vi "16DUT Plot Subvi Ver1.0.vi"(6 "Plot":T1(ring), 7 "No of Rows":i32=10496, 8 "error in (no error)":errorcluster, 9 "WS1050/51":bool=TRUE, 10 "Bank":enum16{"C1", "C2", "C3"}(ring), 11 "file path (dialog if empty)":path) -> (0 "error out":errorcluster, 3 "Delta C_Min Plot":dbl[][](graph) caption="(Y) Multi Plot 2")   [LabVIEW 2012]
uses:
  <vilib>/Utility/file.llb/Read From Spreadsheet File (string).vi
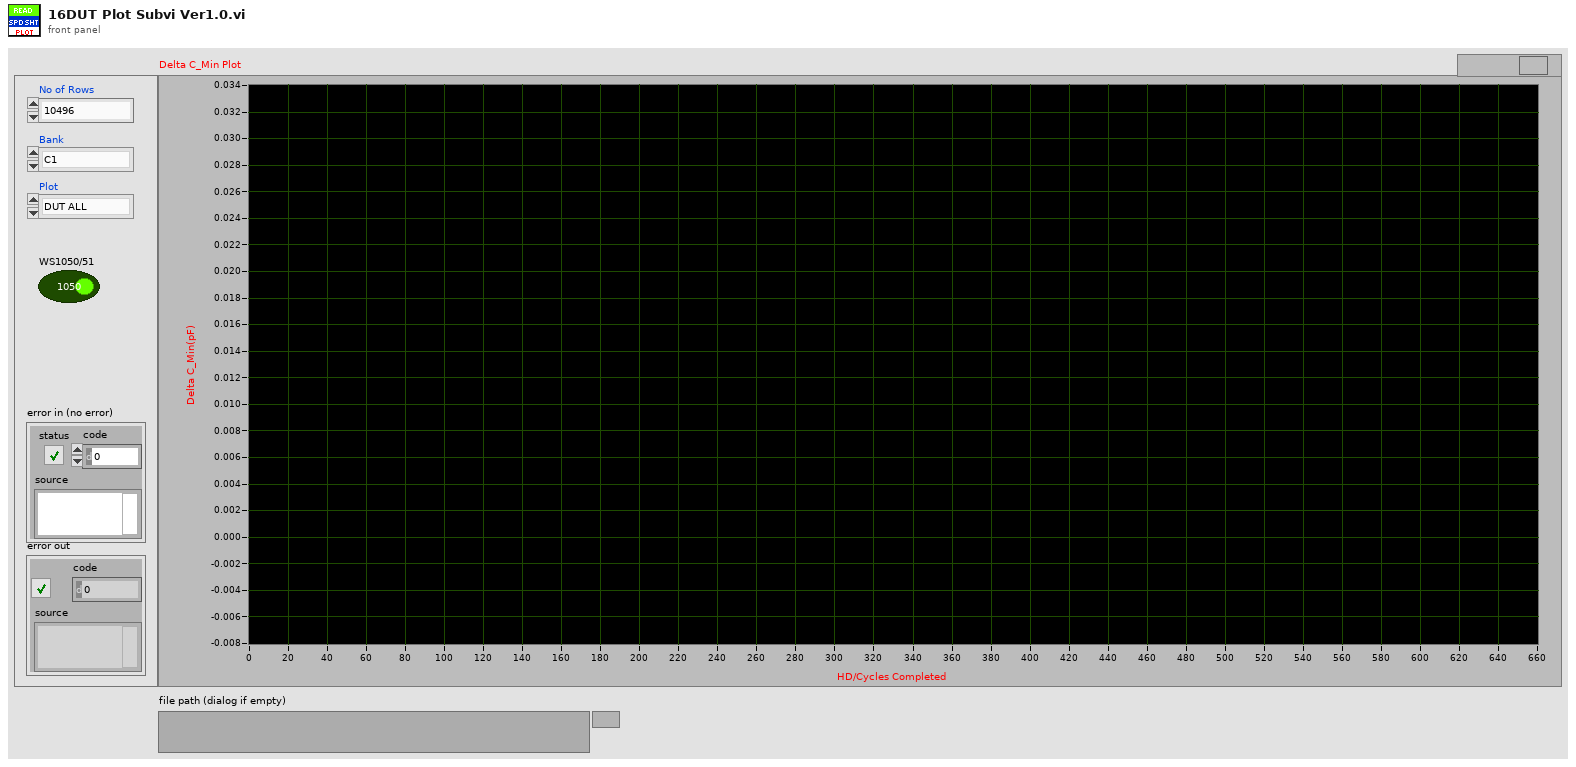
[diagram p1: front panel]
types:
  T1 = enum16{"DUT ALL", "DUT 01", "DUT 02", "DUT 03", "DUT 04", "DUT 05", "DUT 06", "DUT 07", "DUT 08", "DUT 09", "DUT 10", "DUT 11", "DUT 12", "DUT 13", "DUT 14", "DUT 15", "DUT 16"}
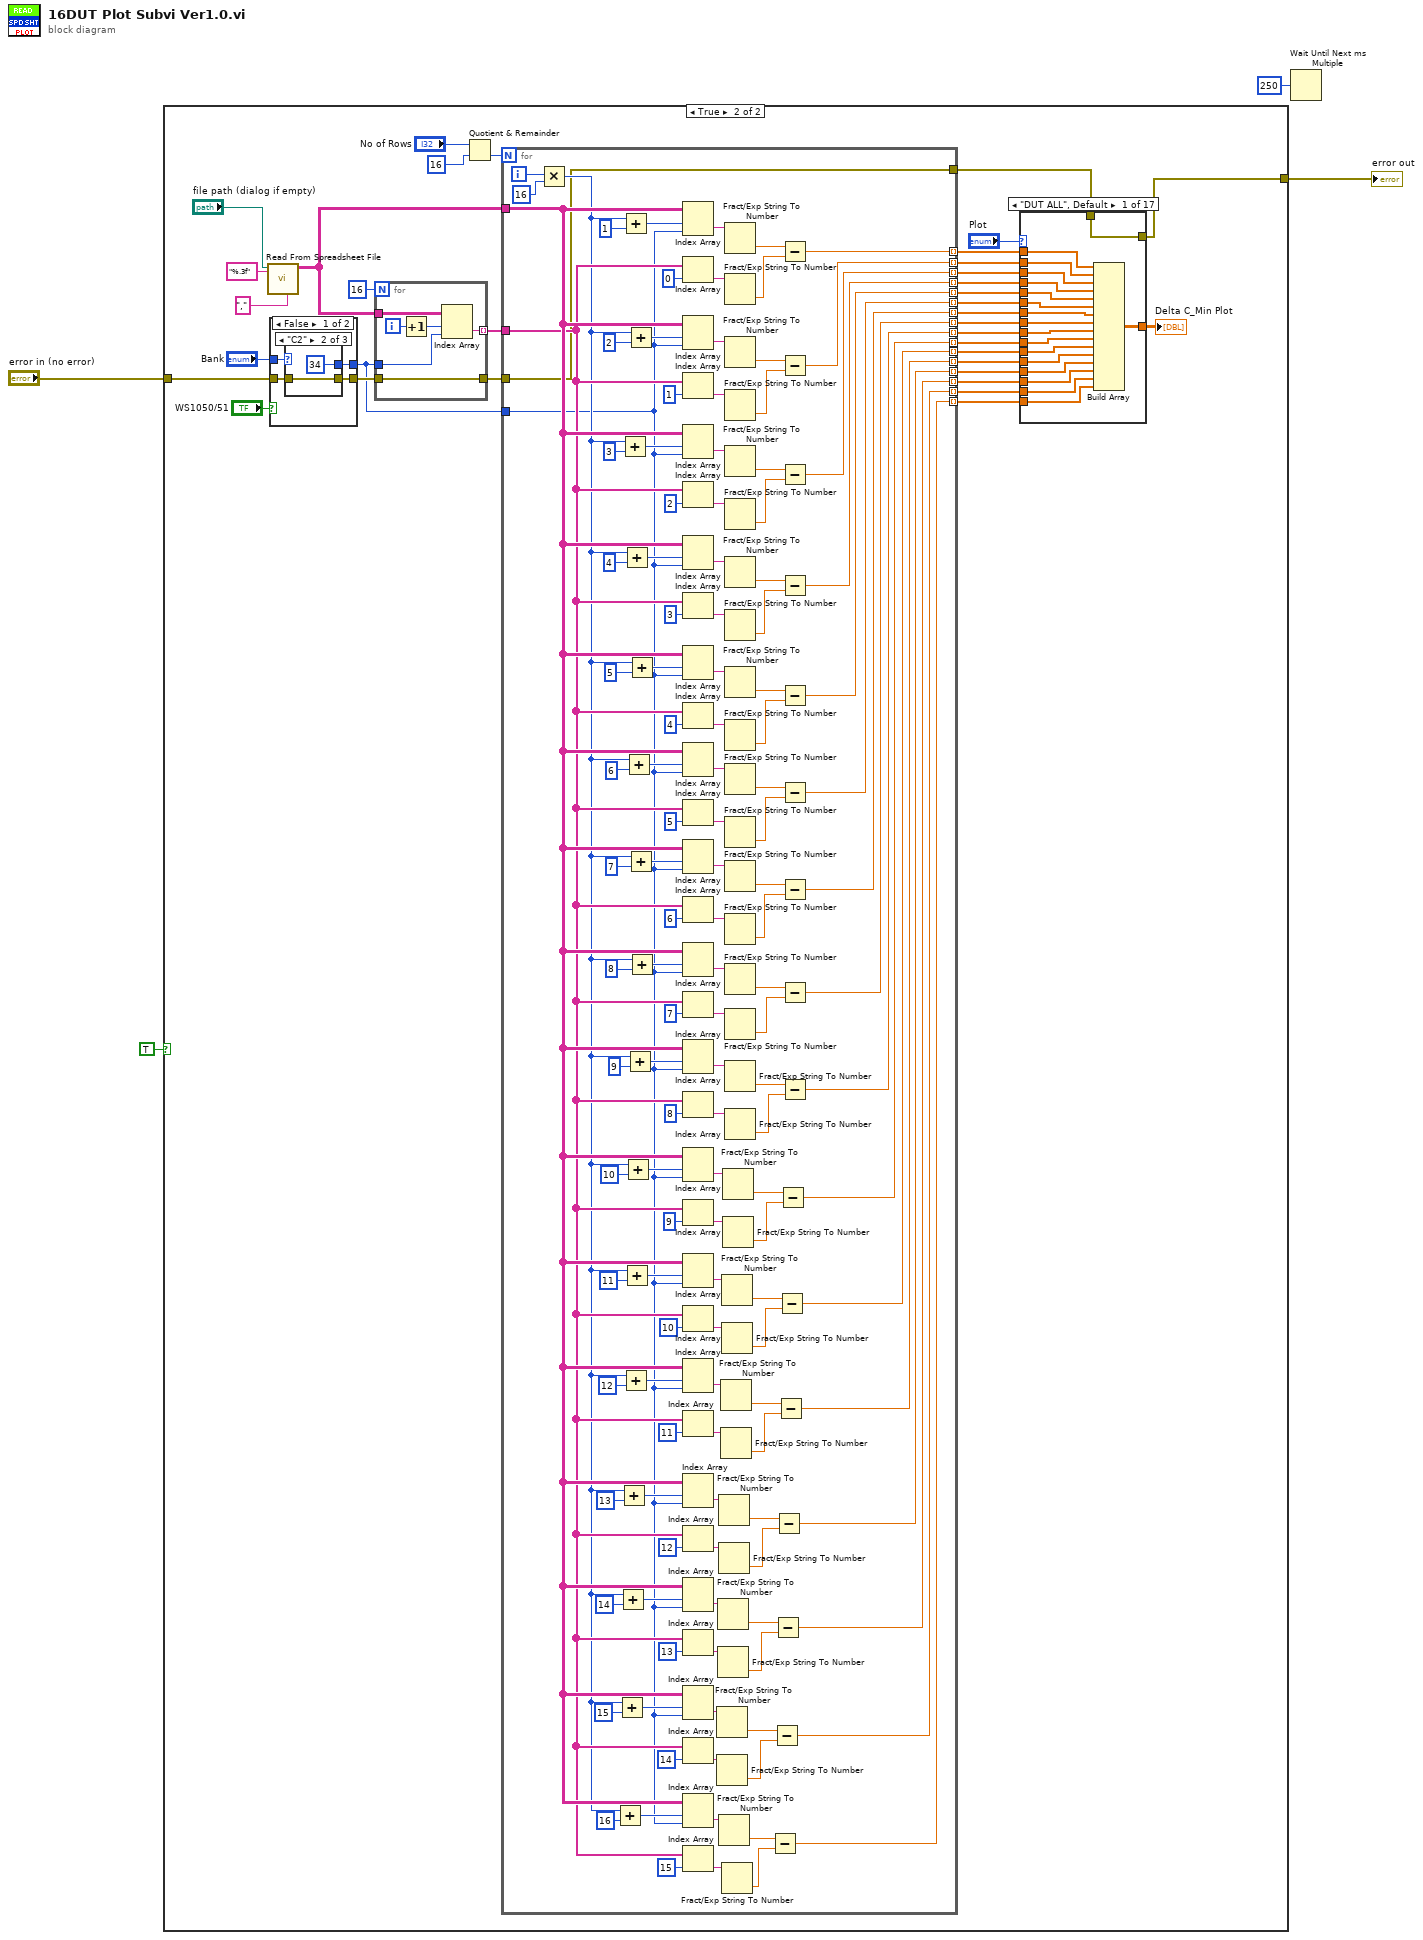
[diagram p0: block diagram]
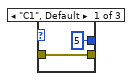
[diagram p3: hidden frame]
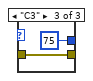
[diagram p4: hidden frame]
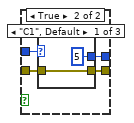
[diagram p5: hidden frame]
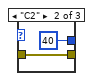
[diagram p6: hidden frame]
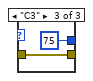
[diagram p7: hidden frame]
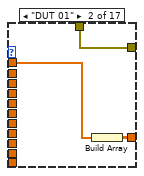
[diagram p8: hidden frame]
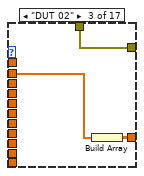
[diagram p9: hidden frame]
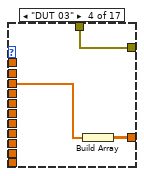
[diagram p10: hidden frame]
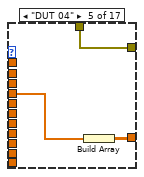
[diagram p11: hidden frame]
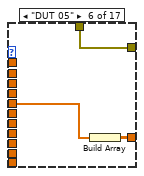
[diagram p12: hidden frame]
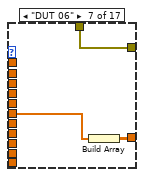
[diagram p13: hidden frame]
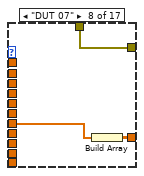
[diagram p14: hidden frame]
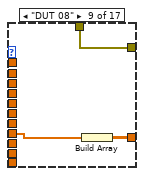
[diagram p15: hidden frame]
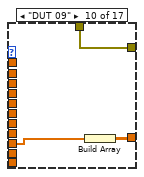
[diagram p16: hidden frame]
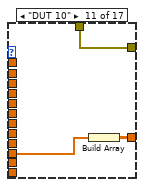
[diagram p17: hidden frame]
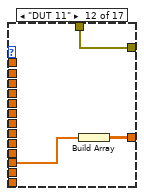
[diagram p18: hidden frame]
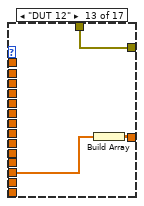
[diagram p19: hidden frame]
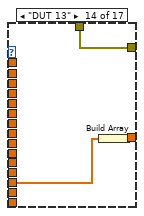
[diagram p20: hidden frame]
diagram:
  n1 = case shown="True" TRUE {
    tunnel: "error in (no error)" -> [w5 w13]
    tunnel: [w5 w8] -> w3
    frame False {
    }
    frame True {
      n2 = call-poly <vilib>:"Read From Spreadsheet File.vi"("delimiter (\\t)"="," ("delimiter (\\t)"), "format (%s)"="%.3f" ("format (%.3f)"), "file path (dialog if empty)"="file path (dialog if empty)") -> ("all rows"=w37:string[][])  [unwired: 4 in, 4 out]
      n3 = case shown="False" "WS1050/51" {
        tunnel: "Bank" -> [w44 w54]
        tunnel: w13 -> [w43 w53]
        tunnel: [w42 w52] -> w10
        tunnel: [w41 w51] -> w6
        frame False {
          n4 = case shown="\"C2\"" w44 {
            tunnel: [5 34 75] -> w41
            tunnel: [w45 w47 w49] -> w42
            tunnel: w43 -> [w45 w47 w49]
            frame "C1", Default {
            }
            frame "C2" {
            }
            frame "C3" {
            }
          }
        }
        frame True {
          n5 = case shown="\"C1\", Default" w54 {
            tunnel: [5 40 75] -> w51
            tunnel: [w55 w57 w59] -> w52
            tunnel: w53 -> [w55 w57 w59]
            frame "C1", Default {
            }
            frame "C2" {
            }
            frame "C3" {
            }
          }
        }
      }
      n6 = for {
        N: 16 -> [_]
        tunnel: w37 -> [w267]
        tunnel: [w266] -> w36 mode=indexing
        tunnel: w6 -> [w262]
        tunnel: [w263] -> w12
        tunnel: w10 -> [w263]
        i -> [w265]
        n7 = Increment(x=w265) -> (x+1=w264:i32)
        n8 = Index Array(array=w267, index (row)=w264, index (col)=w262) -> (element=w266:string)
      }
      n9 = Quotient & Remainder(x="No of Rows", y=16) -> (floor(x/y)=w32:i32)  [unwired: 1 out]
      n10 = for {
        N: w32 -> [_]
        tunnel: w37 -> [w148]
        tunnel: w36 -> [w147]
        tunnel: [w145] -> w30 mode=indexing
        tunnel: [w144] -> w29 mode=indexing
        tunnel: [w143] -> w28 mode=indexing
        tunnel: [w142] -> w27 mode=indexing
        tunnel: [w141] -> w26 mode=indexing
        tunnel: [w140] -> w25 mode=indexing
        tunnel: [w139] -> w24 mode=indexing
        tunnel: [w138] -> w23 mode=indexing
        tunnel: [w137] -> w22 mode=indexing
        tunnel: [w136] -> w21 mode=indexing
        tunnel: [w135] -> w20 mode=indexing
        tunnel: [w134] -> w19 mode=indexing
        tunnel: [w133] -> w18 mode=indexing
        tunnel: [w132] -> w17 mode=indexing
        tunnel: [w131] -> w16 mode=indexing
        tunnel: [w130] -> w15 mode=indexing
        tunnel: w12 -> [w129]
        tunnel: [w129] -> w11
        tunnel: w6 -> [w128]
        i -> [w127]
        n11 = Multiply(x=w127, y=16) -> (x*y=w146:i32)
        n12 = Add(x=w146, y=16) -> (x+y=w153:i32)
        n13 = Add(x=w146, y=15) -> (x+y=w158:i32)
        n14 = Add(x=w146, y=14) -> (x+y=w167:i32)
        n15 = Add(x=w146, y=13) -> (x+y=w172:i32)
        n16 = Add(x=w146, y=3) -> (x+y=w227:i32)
        n17 = Add(x=w146, y=1) -> (x+y=w249:i32)
        n18 = Add(x=w146, y=12) -> (x+y=w181:i32)
        n19 = Add(x=w146, y=4) -> (x+y=w226:i32)
        n20 = Add(x=w146, y=11) -> (x+y=w186:i32)
        n21 = Add(x=w146, y=10) -> (x+y=w195:i32)
        n22 = Add(x=w146, y=6) -> (x+y=w212:i32)
        n23 = Add(x=w146, y=9) -> (x+y=w242:i32)
        n24 = Add(x=w146, y=2) -> (x+y=w246:i32)
        n25 = Add(x=w146, y=7) -> (x+y=w205:i32)
        n26 = Add(x=w146, y=5) -> (x+y=w219:i32)
        n27 = Add(x=w146, y=8) -> (x+y=w199:i32)
        n28 = Index Array(array=w148, index (row)=w249, index (col)=w128) -> (element=w260:string)
        n29 = Index Array(array=w147, index=0) -> (element=w258:string)
        n30 = Index Array(array=w148, index (row)=w246, index (col)=w128) -> (element=w251:string)
        n31 = Index Array(array=w147, index=1) -> (element=w253:string)
        n32 = Index Array(array=w148, index (row)=w227, index (col)=w128) -> (element=w239:string)
        n33 = Index Array(array=w147, index=2) -> (element=w237:string)
        n34 = Index Array(array=w148, index (row)=w226, index (col)=w128) -> (element=w229:string)
        n35 = Index Array(array=w147, index=3) -> (element=w231:string)
        n36 = Index Array(array=w148, index (row)=w219, index (col)=w128) -> (element=w225:string)
        n37 = Index Array(array=w147, index=4) -> (element=w223:string)
        n38 = Index Array(array=w148, index (row)=w212, index (col)=w128) -> (element=w214:string)
        n39 = Index Array(array=w147, index=5) -> (element=w216:string)
        n40 = Index Array(array=w148, index (row)=w205, index (col)=w128) -> (element=w211:string)
        n41 = Index Array(array=w147, index=6) -> (element=w209:string)
        n42 = Index Array(array=w148, index (row)=w199, index (col)=w128) -> (element=w198:string)
        n43 = Index Array(array=w147, index=7) -> (element=w202:string)
        n44 = Index Array(array=w148, index (row)=w242, index (col)=w128) -> (element=w245:string)
        n45 = Index Array(array=w147, index=8) -> (element=w243:string)
        n46 = Index Array(array=w148, index (row)=w195, index (col)=w128) -> (element=w192:string)
        n47 = Index Array(array=w147, index=9) -> (element=w194:string)
        n48 = Index Array(array=w148, index (row)=w186, index (col)=w128) -> (element=w189:string)
        n49 = Index Array(array=w147, index=10) -> (element=w187:string)
        n50 = Index Array(array=w148, index (row)=w181, index (col)=w128) -> (element=w178:string)
        n51 = Index Array(array=w147, index=11) -> (element=w180:string)
        n52 = Index Array(array=w148, index (row)=w172, index (col)=w128) -> (element=w175:string)
        n53 = Index Array(array=w147, index=12) -> (element=w173:string)
        n54 = Index Array(array=w148, index (row)=w167, index (col)=w128) -> (element=w164:string)
        n55 = Index Array(array=w147, index=13) -> (element=w166:string)
        n56 = Index Array(array=w148, index (row)=w158, index (col)=w128) -> (element=w161:string)
        n57 = Index Array(array=w147, index=14) -> (element=w159:string)
        n58 = Index Array(array=w148, index (row)=w153, index (col)=w128) -> (element=w150:string)
        n59 = Index Array(array=w147, index=15) -> (element=w152:string)
        n60 = Fract/Exp String To Number(string=w161) -> (number=w157:dbl)  [unwired: 3 in, 1 out]
        n61 = Fract/Exp String To Number(string=w159) -> (number=w156:dbl)  [unwired: 3 in, 1 out]
        n62 = Fract/Exp String To Number(string=w164) -> (number=w168:dbl)  [unwired: 3 in, 1 out]
        n63 = Fract/Exp String To Number(string=w166) -> (number=w169:dbl)  [unwired: 3 in, 1 out]
        n64 = Fract/Exp String To Number(string=w175) -> (number=w171:dbl)  [unwired: 3 in, 1 out]
        n65 = Fract/Exp String To Number(string=w173) -> (number=w170:dbl)  [unwired: 3 in, 1 out]
        n66 = Fract/Exp String To Number(string=w150) -> (number=w154:dbl)  [unwired: 3 in, 1 out]
        n67 = Fract/Exp String To Number(string=w178) -> (number=w182:dbl)  [unwired: 3 in, 1 out]
        n68 = Fract/Exp String To Number(string=w180) -> (number=w183:dbl)  [unwired: 3 in, 1 out]
        n69 = Fract/Exp String To Number(string=w189) -> (number=w185:dbl)  [unwired: 3 in, 1 out]
        n70 = Fract/Exp String To Number(string=w187) -> (number=w184:dbl)  [unwired: 3 in, 1 out]
        n71 = Fract/Exp String To Number(string=w152) -> (number=w155:dbl)  [unwired: 3 in, 1 out]
        n72 = Fract/Exp String To Number(string=w192) -> (number=w196:dbl)  [unwired: 3 in, 1 out]
        n73 = Fract/Exp String To Number(string=w194) -> (number=w197:dbl)  [unwired: 3 in, 1 out]
        n74 = Fract/Exp String To Number(string=w260) -> (number=w257:dbl)  [unwired: 3 in, 1 out]
        n75 = Fract/Exp String To Number(string=w258) -> (number=w256:dbl)  [unwired: 3 in, 1 out]
        n76 = Fract/Exp String To Number(string=w251) -> (number=w254:dbl)  [unwired: 3 in, 1 out]
        n77 = Fract/Exp String To Number(string=w253) -> (number=w255:dbl)  [unwired: 3 in, 1 out]
        n78 = Fract/Exp String To Number(string=w239) -> (number=w236:dbl)  [unwired: 3 in, 1 out]
        n79 = Fract/Exp String To Number(string=w237) -> (number=w235:dbl)  [unwired: 3 in, 1 out]
        n80 = Fract/Exp String To Number(string=w229) -> (number=w232:dbl)  [unwired: 3 in, 1 out]
        n81 = Fract/Exp String To Number(string=w231) -> (number=w233:dbl)  [unwired: 3 in, 1 out]
        n82 = Fract/Exp String To Number(string=w225) -> (number=w222:dbl)  [unwired: 3 in, 1 out]
        n83 = Fract/Exp String To Number(string=w223) -> (number=w221:dbl)  [unwired: 3 in, 1 out]
        n84 = Fract/Exp String To Number(string=w214) -> (number=w217:dbl)  [unwired: 3 in, 1 out]
        n85 = Fract/Exp String To Number(string=w216) -> (number=w218:dbl)  [unwired: 3 in, 1 out]
        n86 = Fract/Exp String To Number(string=w211) -> (number=w208:dbl)  [unwired: 3 in, 1 out]
        n87 = Fract/Exp String To Number(string=w209) -> (number=w207:dbl)  [unwired: 3 in, 1 out]
        n88 = Fract/Exp String To Number(string=w198) -> (number=w203:dbl)  [unwired: 3 in, 1 out]
        n89 = Fract/Exp String To Number(string=w202) -> (number=w204:dbl)  [unwired: 3 in, 1 out]
        n90 = Fract/Exp String To Number(string=w245) -> (number=w241:dbl)  [unwired: 3 in, 1 out]
        n91 = Fract/Exp String To Number(string=w243) -> (number=w240:dbl)  [unwired: 3 in, 1 out]
        n92 = Subtract(x=w154, y=w155) -> (x-y=w130:dbl)
        n93 = Subtract(x=w157, y=w156) -> (x-y=w131:dbl)
        n94 = Subtract(x=w168, y=w169) -> (x-y=w132:dbl)
        n95 = Subtract(x=w171, y=w170) -> (x-y=w133:dbl)
        n96 = Subtract(x=w182, y=w183) -> (x-y=w134:dbl)
        n97 = Subtract(x=w185, y=w184) -> (x-y=w135:dbl)
        n98 = Subtract(x=w196, y=w197) -> (x-y=w136:dbl)
        n99 = Subtract(x=w257, y=w256) -> (x-y=w145:dbl)
        n100 = Subtract(x=w254, y=w255) -> (x-y=w144:dbl)
        n101 = Subtract(x=w236, y=w235) -> (x-y=w143:dbl)
        n102 = Subtract(x=w232, y=w233) -> (x-y=w142:dbl)
        n103 = Subtract(x=w222, y=w221) -> (x-y=w141:dbl)
        n104 = Subtract(x=w217, y=w218) -> (x-y=w140:dbl)
        n105 = Subtract(x=w208, y=w207) -> (x-y=w139:dbl)
        n106 = Subtract(x=w203, y=w204) -> (x-y=w138:dbl)
        n107 = Subtract(x=w241, y=w240) -> (x-y=w137:dbl)
      }
      n108 = case shown="\"DUT ALL\", Default" "Plot" {
        tunnel: w30 -> [w78 w81 _ _ _ _ _ _ _ _ _ _ _ _ _ _ _]
        tunnel: w29 -> [w77 _ w83 _ _ _ _ _ _ _ _ _ _ _ _ _ _]
        tunnel: w28 -> [w76 _ _ w87 _ _ _ _ _ _ _ _ _ _ _ _ _]
        tunnel: w27 -> [w75 _ _ _ w89 _ _ _ _ _ _ _ _ _ _ _ _]
        tunnel: w26 -> [w74 _ _ _ _ w93 _ _ _ _ _ _ _ _ _ _ _]
        tunnel: w25 -> [w73 _ _ _ _ _ w95 _ _ _ _ _ _ _ _ _ _]
        tunnel: w24 -> [w72 _ _ _ _ _ _ w98 _ _ _ _ _ _ _ _ _]
        tunnel: w23 -> [w71 _ _ _ _ _ _ _ w102 _ _ _ _ _ _ _ _]
        tunnel: w22 -> [w70 _ _ _ _ _ _ _ _ w105 _ _ _ _ _ _ _]
        tunnel: w21 -> [w69 _ _ _ _ _ _ _ _ _ w108 _ _ _ _ _ _]
        tunnel: w20 -> [w68 _ _ _ _ _ _ _ _ _ _ w111 _ _ _ _ _]
        tunnel: w19 -> [w67 _ _ _ _ _ _ _ _ _ _ _ w114 _ _ _ _]
        tunnel: w18 -> [w66 _ _ _ _ _ _ _ _ _ _ _ _ w117 _ _ _]
        tunnel: w17 -> [w65 _ _ _ _ _ _ _ _ _ _ _ _ _ w120 _ _]
        tunnel: w16 -> [w64 _ _ _ _ _ _ _ _ _ _ _ _ _ _ w123 _]
        tunnel: w15 -> [w63 _ _ _ _ _ _ _ _ _ _ _ _ _ _ _ w125]
        tunnel: [w62 w80 w84 w86 w90 w92 w96 w99 w101 w104 w107 w110 w113 w116 w119 w122 w126] -> w14
        tunnel: w11 -> [w61 w79 w82 w85 w88 w91 w94 w97 w100 w103 w106 w109 w112 w115 w118 w121 w124]
        tunnel: [w61 w79 w82 w85 w88 w91 w94 w97 w100 w103 w106 w109 w112 w115 w118 w121 w124] -> w8
        frame "DUT ALL", Default {
          n109 = Build Array(w78, w77, w76, w75, w74, w73, w72, w71, w70, w69, w68, w67, w66, w65, w64, w63) -> (w62:dbl[][])
        }
        frame "DUT 01" {
          n110 = Build Array(w81) -> (w80:dbl[][])
        }
        frame "DUT 02" {
          n111 = Build Array(w83) -> (w84:dbl[][])
        }
        frame "DUT 03" {
          n112 = Build Array(w87) -> (w86:dbl[][])
        }
        frame "DUT 04" {
          n113 = Build Array(w89) -> (w90:dbl[][])
        }
        frame "DUT 05" {
          n114 = Build Array(w93) -> (w92:dbl[][])
        }
        frame "DUT 06" {
          n115 = Build Array(w95) -> (w96:dbl[][])
        }
        frame "DUT 07" {
          n116 = Build Array(w98) -> (w99:dbl[][])
        }
        frame "DUT 08" {
          n117 = Build Array(w102) -> (w101:dbl[][])
        }
        frame "DUT 09" {
          n118 = Build Array(w105) -> (w104:dbl[][])
        }
        frame "DUT 10" {
          n119 = Build Array(w108) -> (w107:dbl[][])
        }
        frame "DUT 11" {
          n120 = Build Array(w111) -> (w110:dbl[][])
        }
        frame "DUT 12" {
          n121 = Build Array(w114) -> (w113:dbl[][])
        }
        frame "DUT 13" {
          n122 = Build Array(w117) -> (w116:dbl[][])
        }
        frame "DUT 14" {
          n123 = Build Array(w120) -> (w119:dbl[][])
        }
        frame "DUT 15" {
          n124 = Build Array(w123) -> (w122:dbl[][])
        }
        frame "DUT 16" {
          n125 = Build Array(w125) -> (w126:dbl[][])
        }
      }
      "Delta C_Min Plot" <- w14
    }
  }
  "error out" <- w3
  n126 = Wait Until Next ms Multiple(millisecond multiple=u32 250) -> ()  [unwired: 1 out]
